vi "Actions.vi"(0 "Magnet":T1, 2 "Array":string[](array[string]), 3 "Data Acq":T2) -> (1 "Abort":bool)   [LabVIEW 2019]
uses:
  Ctl/commands.ctl
  Ctl/Data Acquisition System.ctl
  Ctl/magnet.ctl
panel:
  out "commands":T3=enum."Comments"
  out "valid":bool
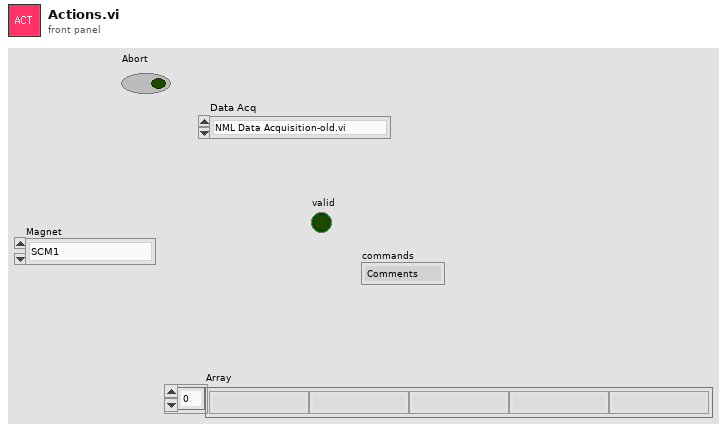
[diagram p1: front panel]
types:
  T1 = typedef "magnet.ctl" = enum16{"SCM1", "SCM2", "SCM3", "SCMX", "Cell8", "Cell9", "Cell12", "Hybrid", "Great Magnet"}
  T2 = typedef "Data Acquisition System.ctl" = enum16{"NML Data Acquisition-old.vi", "NML Data Acquisition-New.vi"}
  T3 = typedef "commands.ctl" = enum16{"Voltage Ramp", "Many Voltage Ramp", "Current Ramp", "Many Current Ramp", "Comments", "Set Field", "Many Set Field", "Abort Sequence", "New-Stop File", "Wait(sec)", "BLM Control", "Many BLM Control", "Stepper Mover", "Many Stepper Mover", "LS336 Ramp Temp", "LakeShore Ramp", "VI Server Control", "LS370 Change Excitation", "Wait Until", "Nothing"}
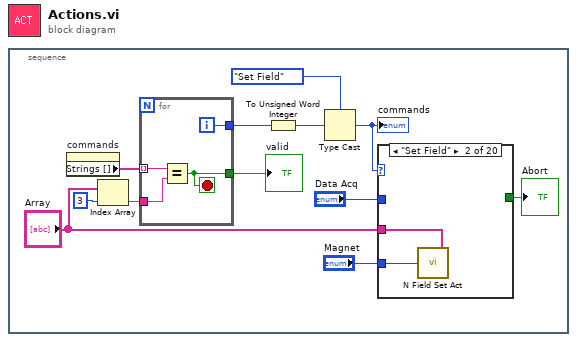
[diagram p0: block diagram]
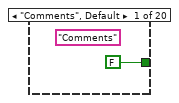
[diagram p2: hidden frame]
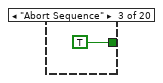
[diagram p3: hidden frame]
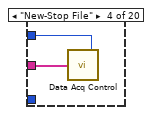
[diagram p4: hidden frame]
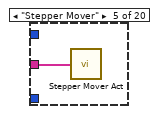
[diagram p5: hidden frame]
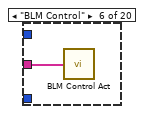
[diagram p6: hidden frame]
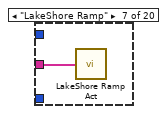
[diagram p7: hidden frame]
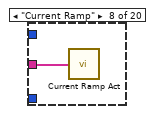
[diagram p8: hidden frame]
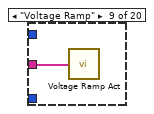
[diagram p9: hidden frame]
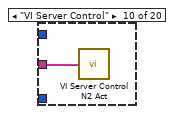
[diagram p10: hidden frame]
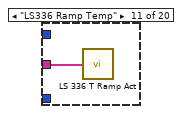
[diagram p11: hidden frame]
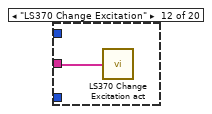
[diagram p12: hidden frame]
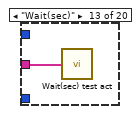
[diagram p13: hidden frame]
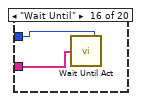
[diagram p16: hidden frame]
diagram:
  n1 = stacked-sequence {
    frame #0 {
      n2 = property on="commands" class="Enum (strict)"() -> ("Strings []"=w5:string[])  [unwired: 2 in, 2 out]
      n3 = Index Array(array="Array", index=3) -> (element=w6:string)
      n4 = for {
        tunnel: w5 -> [w33] mode=indexing
        tunnel: w6 -> [w32]
        tunnel: [w31] -> w11
        tunnel: [w30] -> w12
        i -> [w31]
        stop <- w30 stop-if-true
        n5 = Equal?(x=w33, y=w32) -> (x = y?=w30:bool)
      }
      "valid" <- w12
      n6 = To Unsigned Word Integer(number=w11) -> (unsigned 16bit integer=w10:u16)
      n7 = Type Cast(type=commands."Set Field" ("commands"), x=w10) -> (*(type *) &x=w8:T3)
      "commands" <- w8
      n8 = case shown="\"Set Field\"" w8 {
        tunnel: "Array" -> [_ w15 _ w18 w19 w20 w21 w22 w23 w24 w25 w26 w27 _ _ w29 _ _ _ _]
        tunnel: [FALSE _ TRUE _ _ _ _ _ _ _ _ _ _ _ _ _ _ _ _ _] -> w3
        tunnel: "Data Acq" -> [_ _ _ w17 _ _ _ _ _ _ _ _ _ _ _ w28 _ _ _ _]
        tunnel: "Magnet" -> [_ w14 _ _ _ _ _ _ _ _ _ _ _ _ _ _ _ _ _ _]
        frame "Comments", Default {
          (unwired) "Comments"
        }
        frame "Set Field" {
          n9 = call "N Field Set Act.vi"("command text in"=w15, "Magnet"=w14) -> ()
        }
        frame "Abort Sequence" {
        }
        frame "New-Stop File" {
          n10 = call "Data Acq Control.vi"("Data Acquisition"=w17, "command text in"=w18) -> ()
        }
        frame "Stepper Mover" {
          n11 = call "Stepper Mover Act.vi"("command text in"=w19) -> ()
        }
        frame "BLM Control" {
          n12 = call "BLM Control Act.vi"("command text in"=w20) -> ()
        }
        frame "LakeShore Ramp" {
          n13 = call "LakeShore Ramp Act.vi"("command text in"=w21) -> ()
        }
        frame "Current Ramp" {
          n14 = call "Current Ramp Act.vi"("command text in"=w22) -> ()
        }
        frame "Voltage Ramp" {
          n15 = call "Voltage Ramp Act.vi"("command text in"=w23) -> ()
        }
        frame "VI Server Control" {
          n16 = call "VI Server Control N2 Act.vi"("command text in"=w24) -> ()
        }
        frame "LS336 Ramp Temp" {
          n17 = call "LS 336 T Ramp Act.vi"("command text in"=w25) -> ()
        }
        frame "LS370 Change Excitation" {
          n18 = call "LS370 Change Excitation act.vi"("command text in"=w26) -> ()
        }
        frame "Wait(sec)" {
          n19 = call "Wait(sec) test act.vi"("command text in"=w27) -> ()
        }
        frame "Many BLM Control" {
        }
        frame "Many Stepper Mover" {
        }
        frame "Wait Until" {
          n20 = call "Wait Until Act.vi"("Data Acq"=w28, "command text in"=w29) -> ()
        }
        frame "Nothing" {
        }
        frame "Many Voltage Ramp" {
        }
        frame "Many Current Ramp" {
        }
        frame "Many Set Field" {
        }
      }
      "Abort" <- w3
    }
  }
